vi "globals.vi"() -> ()   [LabVIEW 2017]
panel:
  out "Match Timer":dbl
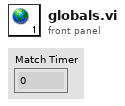
[diagram p1: front panel]
diagram:
